vi "Set Transfer Type.vi"(8 "error in":errorcluster, 10 "transfer type":T1, 11 "label ref in":T2 format="%.0x") -> (0 "error out":errorcluster, 3 "label ref out":T2 format="%.0x")   [LabVIEW 2020, in "AIM ARINC 429 Scripting.lvlib"]
uses:
  <vilib>/NI VeriStand/Custom Device API/Custom Device Item Ref.ctl
  Shared/Transfer Type.ctl
  AIM/Constants.vi
  <vilib>/NI VeriStand/Custom Device API/Set Item Property (U16).vi
  AIM/AIM ARINC 429 Scripting.lvlib
  <vilib>/NI VeriStand/Custom Device API/Custom Device API.lvlib
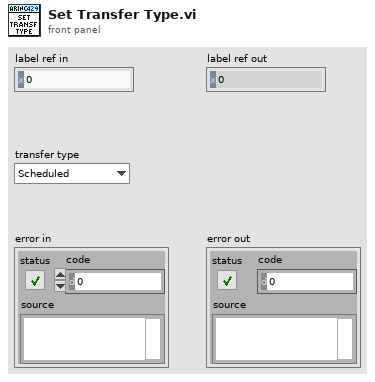
[diagram p1: front panel]
types:
  T1 = typedef "Transfer Type.ctl" = enum16{"Scheduled", "Acyclic", "Block", "Strobe"}
  T2 = typedef "Custom Device API.lvlib/Custom Device Item Ref.ctl" = u64
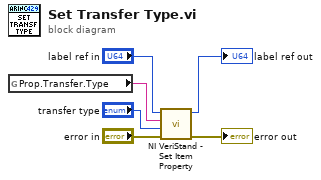
[diagram p0: block diagram]
diagram:
  n1 = global read "Constants.vi" "Prop.Transfer.Type"() -> (w4:string)
  n2 = call-poly <vilib>:"NI VeriStand - Set Item Property.vi"("error in (no error)"="error in", "Value"="transfer type", "Property Name"=w4, "Item Ref in"="label ref in") -> ("error out"=→"error out":errorcluster, "Item Ref out"=→"label ref out":T2)  [unwired: 5 in, 1 out]
